vi "NewLot.vi"(7 "FilePath":path, 8 "error in (no error)":errorcluster, 9 "Type":string, 10 "Wafer ID":string, 11 "LotData in":refnum<class "LotData.lvclass">) -> (0 "error out":errorcluster, 3 "LotData out":refnum<class "LotData.lvclass">)   [LabVIEW 2012, in "LotData.lvclass"]
uses:
  LotData.lvclass
  Controls/TestData.ctl
  Controls/Measurement.ctl
  Controls/LotData_Current.ctl
  LotData.lvclass/LotData.ctl
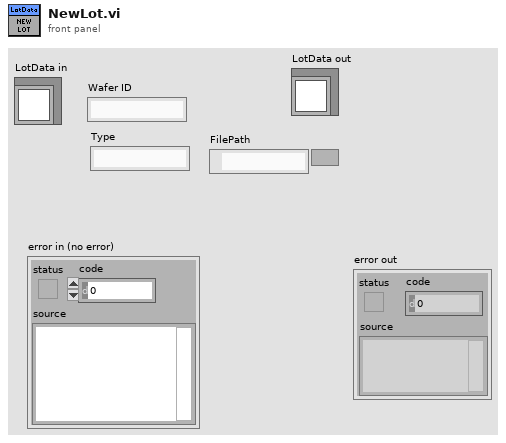
[diagram p1: front panel]
types:
  T1 = cluster{"Area":string, "Wavelength":dbl[], "EL Spectrum":dbl[]}
  T2 = typedef "TestData.ctl" = cluster{"20mA Data":T3, "50mA Data ":T3}
  T3 = typedef "Measurement.ctl" = cluster{"Area":string, "Pad":string, "Current,mA":dbl, "Power":dbl, "WL":dbl, "Voltage":dbl, "Knee Current":dbl, "Reverse":dbl}
  T4 = typedef "LotData.lvclass/LotData_Current.ctl" = cluster{"area":i32, "Data":cluster{"wl":dbl, "power":dbl, "voltage":dbl, "knee":dbl, "reverse":dbl}}
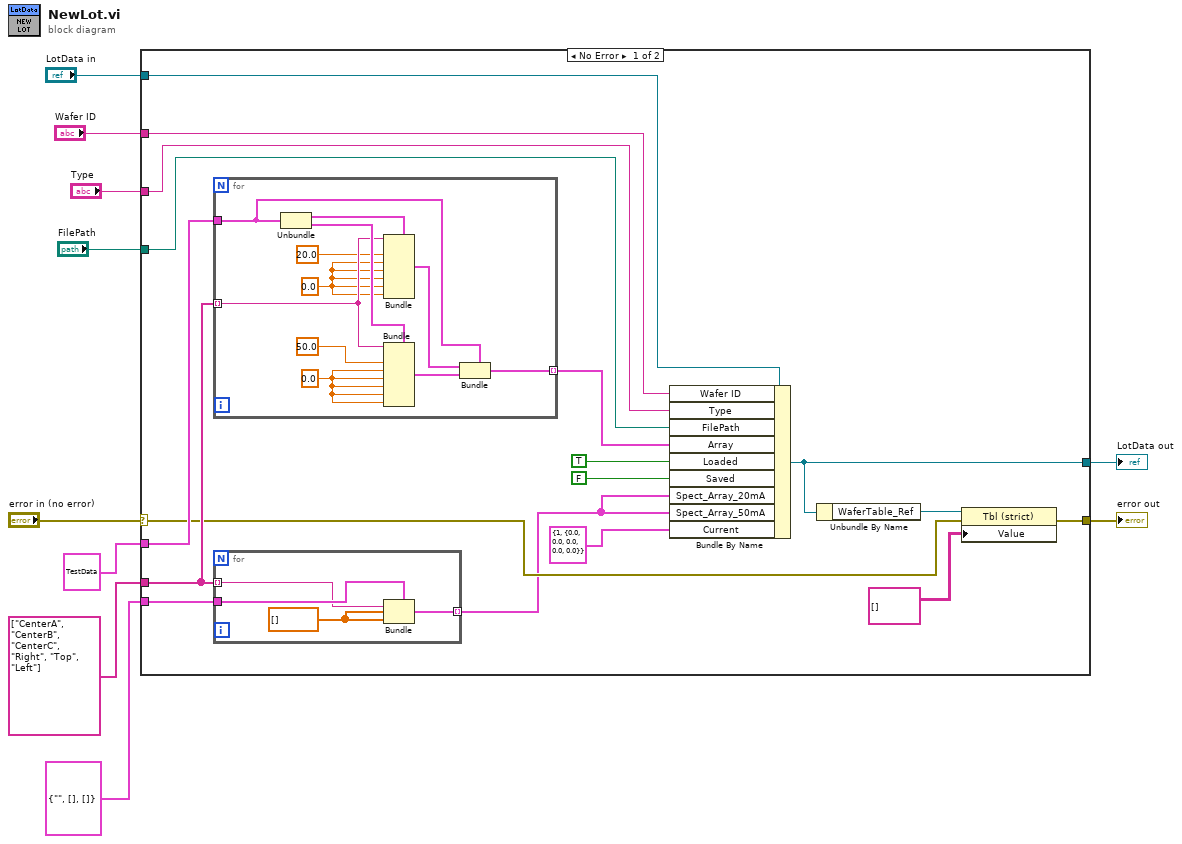
[diagram p0: block diagram]
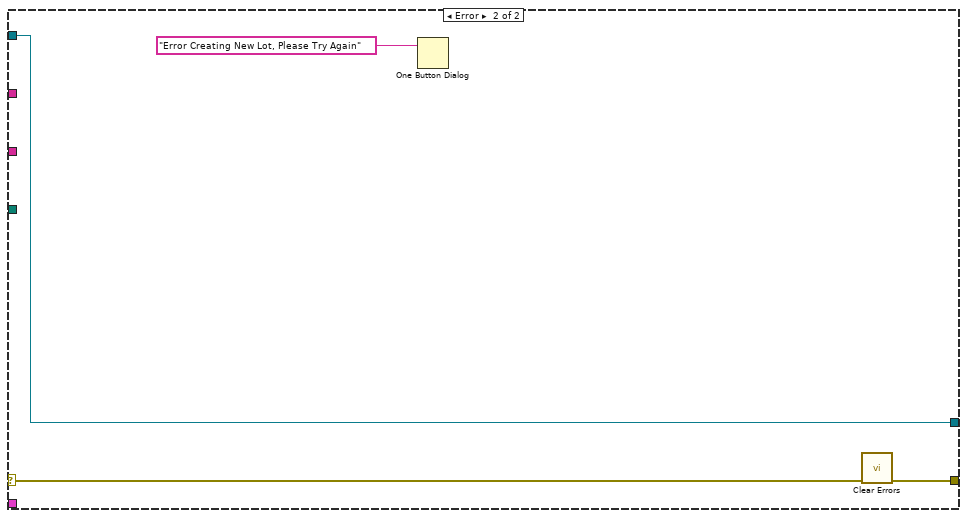
[diagram p2: hidden frame]
diagram:
  n1 = case shown="No Error" "error in (no error)" {
    selector: "error in (no error)" -> [w15 w44]
    tunnel: [w18 w43] -> w9
    tunnel: "LotData in" -> [w11 w46]
    tunnel: "Wafer ID" -> [w27 _]
    tunnel: "Type" -> [w14 _]
    tunnel: "FilePath" -> [w26 _]
    tunnel: T2 {"20mA Data"={"Area"="", "Pad"="", "Current,mA"=0.0, "Power"=0.0, "WL"=0.0, "Voltage"=0.0, "Knee Current"=0.0, "Reverse"=0.0}, "50mA Data "={"Area"="", "Pad"="", "Current,mA"=0.0, "Power"=0.0, "WL"=0.0, "Voltage"=0.0, "Knee Current"=0.0, "Reverse"=0.0}} ("TestData") -> [w25 _]
    tunnel: string[] ["CenterA", "CenterB", "CenterC", "Right", "Top", "Left"] -> [w17 _]
    tunnel: [w19 w46] -> w4
    tunnel: T1 {"Area"="", "Wavelength"=[], "EL Spectrum"=[]} ("Spect") -> [w16 _]
    frame No Error {
      n2 = for {
        tunnel: w25 -> [w39]
        tunnel: w17 -> [w40] mode=indexing
        tunnel: [w36] -> w24 mode=indexing
        w34 = 0.0 ("Power")
        w33 = 0.0 ("Power")
        n3 = Unbundle(w39) -> ("20mA Data"=w42:T3, "50mA Data"=w41:T3)
        n4 = Bundle(cluster=w42, "Area"=w40, "Current,mA"=20.0, "Power"=w33, "WL"=w33, "Voltage"=w33, "Knee Current"=w33, "Reverse"=w33) -> (w38:T3)  [unwired: 1 in]
        n5 = Bundle(cluster=w41, "Area"=w40, "Current,mA"=50.0, "Power"=w34, "WL"=w34, "Voltage"=w34, "Knee Current"=w34, "Reverse"=w34) -> (w37:T3)  [unwired: 1 in]
        n6 = Bundle(cluster=w39, "20mA Data"=w38, "50mA Data"=w37) -> (w36:T2)
      }
      n7 = for {
        tunnel: w17 -> [w30] mode=indexing
        tunnel: w16 -> [w31]
        tunnel: [w28] -> w13 mode=indexing
        w29 = dbl[] [] ("Wavelength")
        n8 = Bundle(cluster=w31, "Area"=w30, "Wavelength"=w29, "EL Spectrum"=w29) -> (w28:T1)
      }
      n9 = Bundle By Name(cluster=w11, "Wafer ID"=w27, "Type"=w14, "FilePath"=w26, "Array"=w24, "Loaded"=TRUE, "Saved"=FALSE, "Spect_Array_20mA"=w13, "Spect_Array_50mA"=w13, "Current"=T4 {"area"=1, "Data"={"wl"=0.0, "power"=0.0, "voltage"=0.0, "knee"=0.0, "reverse"=0.0}}) -> (w19:refnum<class "LotData.lvclass">)
      n10 = Unbundle By Name(w19) -> ("WaferTable_Ref"=w20:refnum<vi>)
      n11 = property class="Tbl (strict)"(reference=w20, error in=w15, "Value"=string[][] []) -> (error out=w18:errorcluster)  [unwired: 1 out]
    }
    frame Error {
      n12 = One Button Dialog(message="Error Creating New Lot, Please Try Again") -> ()  [unwired: 1 in, 1 out]
      n13 = call <vilib>:"Clear Errors.vi"("error in (no error)"=w44) -> ("error out"=w43:errorcluster)  [unwired: 6 in]
    }
  }
  "error out" <- w9
  "LotData out" <- w4
